vi "Set Callback On Play Metadata.vi"(10 "OnPlayMetadata":cluster{}, 11 "index":u16) -> (3 "function return":i32)   [LabVIEW 2025, in "ExtremelyEpicImagerIPC2.lvlib"]
doc: "IMAGERIPC_API HRESULT WINAPI SetCallback_OnPlayMetadata(WORD index, fpOnBufferSend OnPlayMetadata);"
uses:
  ExtremelyEpicImagerIPC2.lvlib
  ImagerIPC2.dll
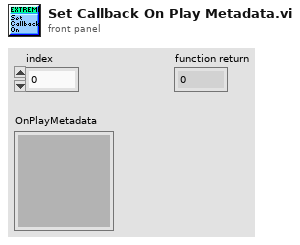
[diagram p1: front panel]
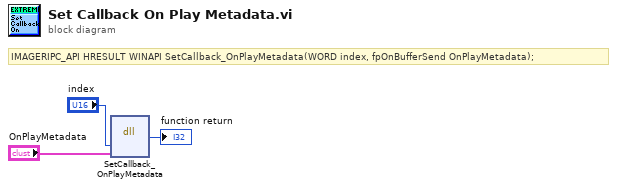
[diagram p0: block diagram]
diagram:
  # "IMAGERIPC_API HRESULT WINAPI SetCallback_OnPlayMetadata(WORD index, fpOnBufferSend OnPlayMetadata);"
  n1 = dll-call lib="C:/Users/mayhe/OneDrive/Documents/GitHub/In-situ-monitoring-of-powder-bed-fusion-additive-manufacturing/system_development/Orichalcum/v0.2/Software_design/thermal-camera/VI/Connect SDK/ImagerIPC2.*" fn="SetCallback_OnPlayMetadata"("index"="index", "OnPlayMetadata"="OnPlayMetadata") -> (→"function return":i32)  [unwired: 5 in, 2 out]
